vi "SIM Init Special Solver (vector).vi"(4 "Output":dbl[](array[numeric]), 5 "State Index":i32, 6 "State Name":string, 7 "Simulation data":T1={"continuous integrator"=enum."RK 1 (Euler)", "initial time"=0.0, "final time"=0.0, "step size"=0.0, "proposed step size"=0.0, "max step size"=0.0, "min step size"=0.0, "discrete time step"=0.0, "max step ratio"=0.0, "Diag Eval Stage"=enum."Init", "Substep Index"=0, "Timestep Index"=0.0, "simulation time"=0.0, "current timestep base"=0.0, "proposed step time"=0.0, "absolute tolerance"=0.0, "relative tolerance"=0.0, "step accepted?"=FALSE, "step complete?"=FALSE, "Halt?"=FALSE, "reset integrator?"=FALSE, "machine epsilon"=0.0, "min float"=0.0, "error"={"status"=FALSE, "code"=0, "source"=""}, "Method Order"=0, "Finished Late [i-1]"=FALSE, "Discrete step?"=FALSE, "NaN and Inf check?"=FALSE, "Final Timestep Index"=0.0, "(maj+disc)or(init)?"=FALSE, "Full Solver Reset"=TRUE, "Execution Mode"=enum."Simulate to Completion", "check vector sizes?"=FALSE, "solver handles zc?"=FALSE, "Simulation Registry"={"Current Idx"=0, "Node Tags"=[], "Node Headers"=[], "Node Data"=[], "Cont State data"={"inputs"=[], "outputs"=[], "reset"=[], "lower limits"=[], "upper limits"=[], "limit types"=[], "reset types"=[], "initial conditions"=[], "reset I.C."=[], "limited?"=[], "State Names"=[]}, "DiscreteInfo"={"tick period (sec)"=0.0, "time (ticks)"=0, "fire?"=[], "registry"={"period (sec)"=[], "skew (sec)"=[], "period (tick)"=[], "skew (tick)"=[]}, "discrete \nblocks?"=FALSE, "steps per tick"=0.0, "steps to tick"=0.0, "discrete \ntick?"=FALSE}, "Disc State data"={"Disc States"=[], "State Names"=[]}, "Registry Error"={"Error Block ID"=0, "code"=0}, "ZC Indices"=[]}, "variable step solver?"=FALSE, "First Substep?"=FALSE, "Continuous States?"=FALSE} {"min float" format="%.1e"; "proposed step size" format="%.1e"; "proposed step time" format="%.1e"; "max step ratio" format="%.1e"; "min step size" format="%.1e"; "machine epsilon" format="%.1e"; "discrete time step" format="%.1e"; "max step size" format="%.1e"; "current timestep base" format="%.1e"; "final time" format="%.1e"; "simulation time" format="%.1e"; "relative tolerance" format="%.1e"; "absolute tolerance" format="%.1e"; "Substep Index" format="%.1e"; "step size" format="%.1e"; "initial time" format="%.1e"}) -> (0 "Modified Output":dbl[](array[numeric]), 3 "Simulation data out":T1={"continuous integrator"=enum."RK 1 (Euler)", "initial time"=0.0, "final time"=0.0, "step size"=0.0, "proposed step size"=0.0, "max step size"=0.0, "min step size"=0.0, "discrete time step"=0.0, "max step ratio"=0.0, "Diag Eval Stage"=enum."Init", "Substep Index"=0, "Timestep Index"=0.0, "simulation time"=0.0, "current timestep base"=0.0, "proposed step time"=0.0, "absolute tolerance"=0.0, "relative tolerance"=0.0, "step accepted?"=FALSE, "step complete?"=FALSE, "Halt?"=FALSE, "reset integrator?"=FALSE, "machine epsilon"=0.0, "min float"=0.0, "error"={"status"=FALSE, "code"=0, "source"=""}, "Method Order"=0, "Finished Late [i-1]"=FALSE, "Discrete step?"=FALSE, "NaN and Inf check?"=FALSE, "Final Timestep Index"=0.0, "(maj+disc)or(init)?"=FALSE, "Full Solver Reset"=TRUE, "Execution Mode"=enum."Simulate to Completion", "check vector sizes?"=FALSE, "solver handles zc?"=FALSE, "Simulation Registry"={"Current Idx"=0, "Node Tags"=[], "Node Headers"=[], "Node Data"=[], "Cont State data"={"inputs"=[], "outputs"=[], "reset"=[], "lower limits"=[], "upper limits"=[], "limit types"=[], "reset types"=[], "initial conditions"=[], "reset I.C."=[], "limited?"=[], "State Names"=[]}, "DiscreteInfo"={"tick period (sec)"=0.0, "time (ticks)"=0, "fire?"=[], "registry"={"period (sec)"=[], "skew (sec)"=[], "period (tick)"=[], "skew (tick)"=[]}, "discrete \nblocks?"=FALSE, "steps per tick"=0.0, "steps to tick"=0.0, "discrete \ntick?"=FALSE}, "Disc State data"={"Disc States"=[], "State Names"=[]}, "Registry Error"={"Error Block ID"=0, "code"=0}, "ZC Indices"=[]}, "variable step solver?"=FALSE, "First Substep?"=FALSE, "Continuous States?"=FALSE} {"min float" format="%.1e"; "proposed step size" format="%.1e"; "proposed step time" format="%.1e"; "max step ratio" format="%.1e"; "min step size" format="%.1e"; "machine epsilon" format="%.1e"; "discrete time step" format="%.1e"; "max step size" format="%.1e"; "current timestep base" format="%.1e"; "final time" format="%.1e"; "simulation time" format="%.1e"; "relative tolerance" format="%.1e"; "absolute tolerance" format="%.1e"; "Substep Index" format="%.1e"; "step size" format="%.1e"; "initial time" format="%.1e"})   [LabVIEW 2017]
uses:
  <vilib>/Simulation/Implementation/Shared/SIM simulation data.ctl
  <vilib>/Simulation/Implementation/Shared/SIM integration method.ctl
  <vilib>/Simulation/Implementation/Shared/SIM diagram eval stage.ctl
  <vilib>/Simulation/Implementation/Shared/SIMSCR Execution Mode.ctl
  <vilib>/Simulation/Implementation/Shared/SIM Registry.llb/SIM Simulation Registry.ctl
  <vilib>/Simulation/Implementation/Shared/SIM Registry.llb/SIM Registry Node Header.ctl
  <vilib>/Simulation/Implementation/Shared/SIM Registry.llb/SIM Registry Node Record.ctl
  <vilib>/Simulation/Implementation/Shared/SIM trigger type.ctl
  <vilib>/Simulation/Implementation/Shared/SIM solver state data.ctl
  <vilib>/Simulation/Implementation/Shared/SIM limit type.ctl
  <vilib>/Simulation/Implementation/Shared/SIM discrete data.ctl
  <vilib>/Simulation/Implementation/Shared/SIM Discrete state data.ctl
  <vilib>/Simulation/Implementation/Shared/SIM Registry.llb/SIM Simulation Registry Error.ctl
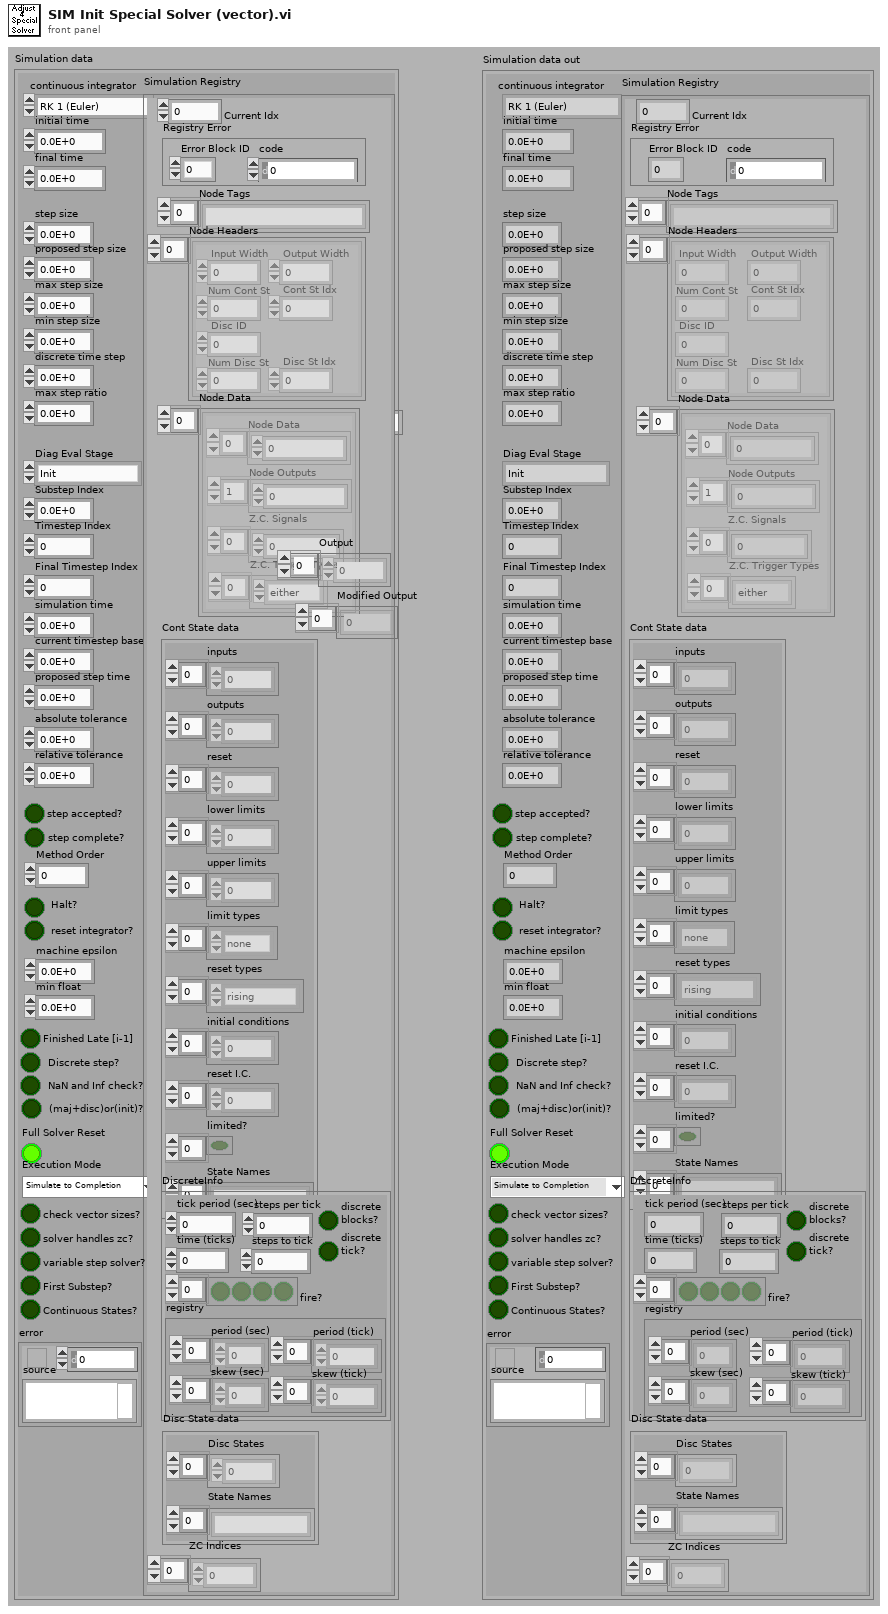
[diagram p1: front panel]
types:
  T1 = typedef "SIM simulation data.ctl" = cluster{"continuous integrator":T2, "initial time":dbl, "final time":dbl, "step size":dbl, "proposed step size":dbl, "max step size":dbl, "min step size":dbl, "discrete time step":dbl, "max step ratio":dbl, "Diag Eval Stage":T3, "Substep Index":i32, "Timestep Index":dbl, "simulation time":dbl, "current timestep base":dbl, "proposed step time":dbl, "absolute tolerance":dbl, "relative tolerance":dbl, "step accepted?":bool, "step complete?":bool, "Halt?":bool, "reset integrator?":bool, "machine epsilon":dbl, "min float":dbl, "error":errorcluster, "Method Order":u32, "Finished Late [i-1]":bool, "Discrete step?":bool, "NaN and Inf check?":bool, "Final Timestep Index":dbl, "(maj+disc)or(init)?":bool, "Full Solver Reset":bool, "Execution Mode":T4, "check vector sizes?":bool, "solver handles zc?":bool, "Simulation Registry":T5, "variable step solver?":bool, "First Substep?":bool, "Continuous States?":bool}
  T2 = typedef "SIM integration method.ctl" = enum16{"RK 1 (Euler)", "Linearizer", "State Query", "Trim Eval", "Adams", "RK 3", "RK 4", "RK 45", "BDF", "RK 2", "RK 23", "Rosenbrock", "Discrete States Only"}
  T3 = typedef "SIM diagram eval stage.ctl" = enum16{"Init", "Minor Substep", "Major Substep", "Final"}
  T4 = typedef "SIMSCR Execution Mode.ctl" = enum16{"Simulate to Completion", "Single Time-Step Simulation (Fixed Step Only)"}
  T5 = typedef "SIM Simulation Registry.ctl" = cluster{"Current Idx":i32, "Node Tags":string[], "Node Headers":T6[], "Node Data":T7[], "Cont State data":T9, "DiscreteInfo":T11, "Disc State data":T12, "Registry Error":T13, "ZC Indices":i32[]}
  T6 = typedef "SIM Registry Node Header.ctl" = cluster{"Input Width":i32, "Disc ID":i32, "Num Cont St":i32, "Cont St Idx":i32, "Num Disc St":i32, "Disc St Idx":i32, "Output Width":i32}
  T7 = typedef "SIM Registry Node Record.ctl" = cluster{"Node Data":dbl[], "Node Outputs":dbl[], "Z.C. Signals":dbl[], "Z.C. Trigger Types":T8[]}
  T8 = typedef "SIM trigger type.ctl" = enum16{"rising", "falling", "either", "none"}
  T9 = typedef "SIM solver state data.ctl" = cluster{"inputs":dbl[], "outputs":dbl[], "reset":dbl[], "lower limits":dbl[], "upper limits":dbl[], "limit types":T10[], "reset types":T8[], "initial conditions":dbl[], "reset I.C.":dbl[], "limited?":bool[], "State Names":string[]}
  T10 = typedef "SIM limit type.ctl" = enum16{"upper", "lower", "both", "none"}
  T11 = typedef "SIM discrete data.ctl" = cluster{"tick period (sec)":dbl, "time (ticks)":i32, "fire?":bool[], "registry":cluster{"period (sec)":dbl[], "skew (sec)":dbl[], "period (tick)":i32[], "skew (tick)":i32[]}, "discrete \nblocks?":bool, "steps per tick":dbl, "steps to tick":dbl, "discrete \ntick?":bool}
  T12 = typedef "SIM Discrete state data.ctl" = cluster{"Disc States":dbl[], "State Names":string[]}
  T13 = typedef "SIM Simulation Registry Error.ctl" = cluster{"Error Block ID":i32, "code":i32}
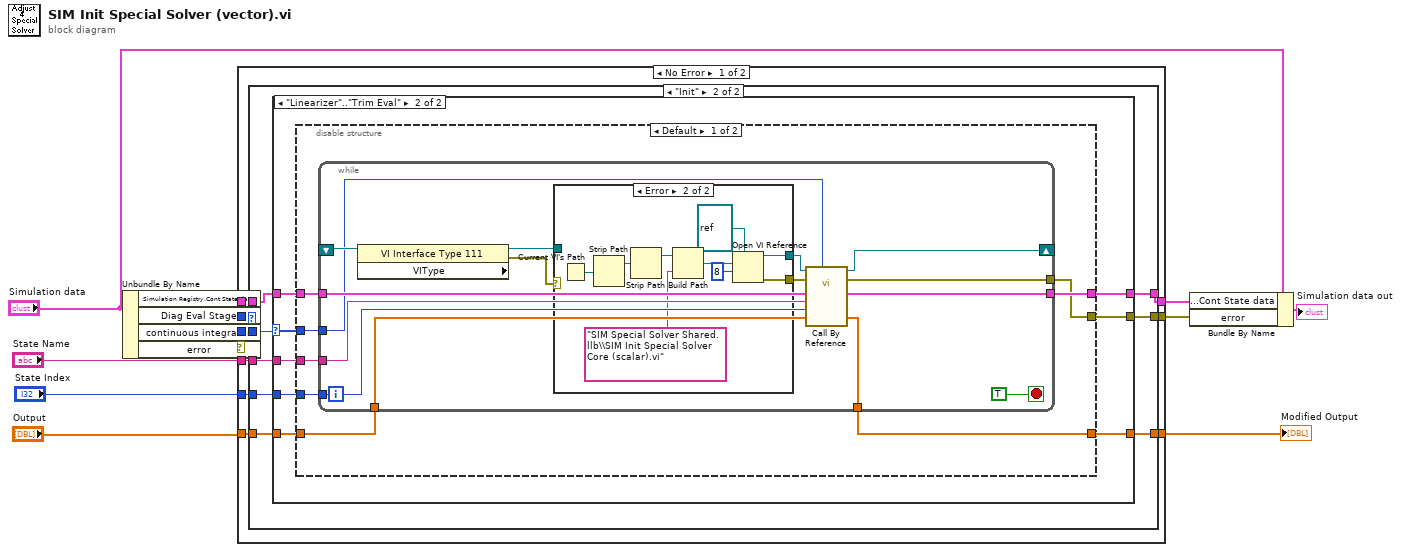
[diagram p0: block diagram]
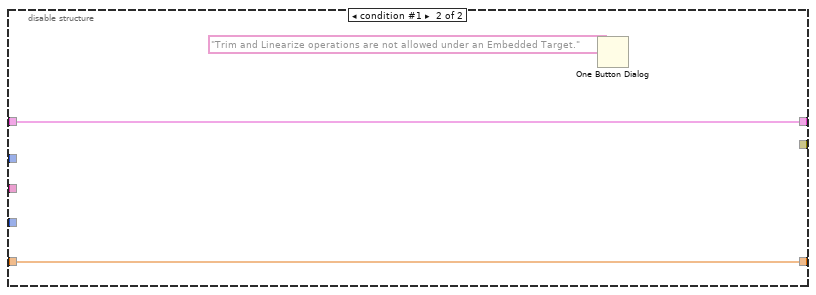
[diagram p5: hidden frame]
diagram:
  n1 = Unbundle By Name("Simulation data") -> ("Simulation Registry.Cont State data"=w10:T9, "Diag Eval Stage"=w12:T3, "continuous integrator"=w11:T2, "error"=w8:errorcluster)
  n2 = case shown="No Error" w8 {
    selector: w8 -> [_ w79]
    tunnel: "State Name" -> [w21 _]
    tunnel: "State Index" -> [w20 _]
    tunnel: w12 -> [w19 _]
    tunnel: "Output" -> [w18 _]
    tunnel: [w17 _] -> w1
    tunnel: w11 -> [w16 _]
    tunnel: w10 -> [w15 w80]
    tunnel: [w14 w80] -> w9
    tunnel: [w13 w79] -> w7
    frame No Error {
      n3 = case shown="\"Init\"" w19 {
        tunnel: w21 -> [_ w28]
        tunnel: w20 -> [_ w29]
        tunnel: w15 -> [w23 w31]
        tunnel: [w23 w27] -> w14
        tunnel: w18 -> [w22 w30]
        tunnel: [w22 w26] -> w17
        tunnel: w16 -> [_ w25]
        tunnel: [_ w24] -> w13
        frame Default {
        }
        frame "Init" {
          n4 = case shown="\"Linearizer\"..\"Trim Eval\"" w25 {
            selector: w25 -> [_ w35]
            tunnel: w31 -> [w32 w41]
            tunnel: w30 -> [w33 w40]
            tunnel: w29 -> [_ w36]
            tunnel: w28 -> [_ w39]
            tunnel: [w32 w37] -> w27
            tunnel: [w33 w38] -> w26
            tunnel: [_ w34] -> w24
            frame Default {
            }
            frame "Linearizer".."Trim Eval" {
              n5 = disable-structure shown="Default" {
                disable-tunnel: w41 -> [w49 w78]
                disable-tunnel: w40 -> [w48 w77]
                disable-tunnel: w39 -> [w47 _]
                disable-tunnel: [w46 w77] -> w38
                disable-tunnel: [w45 w78] -> w37
                disable-tunnel: w36 -> [w44 _]
                disable-tunnel: w35 -> [w43 _]
                disable-tunnel: [w42 _] -> w34
                frame condition #0 (active) {
                  n6 = while {
                    tunnel: w49 -> [w60]
                    tunnel: w48 -> [w57]
                    tunnel: w47 -> [w59]
                    tunnel: [w56] -> w46
                    tunnel: [w52] -> w45
                    tunnel: w44 -> [w58]
                    shift-right: [w55] -> _
                    shift-left: _ -> [w63]
                    tunnel: w43 -> [w51]
                    tunnel: [w50] -> w42
                    stop <- TRUE stop-if-true
                    n7 = property class="VI Interface Type 111" props=["VIType"](reference=w63) -> (reference out=w54:refnum<vi>, error out=w61:errorcluster)  [unwired: 1 in, 1 out]
                    n8 = case shown="Error" w61 {
                      selector: w61 -> [w66 _]
                      tunnel: [w66 w75] -> w64
                      tunnel: [w65 w69] -> w53
                      tunnel: w54 -> [w65 _]
                      frame No Error {
                      }
                      frame Error {
                        n9 = Current VI's Path() -> (path=w74:path)
                        n10 = Strip Path(path=w74) -> (stripped path=w68:path)  [unwired: 1 out]
                        n11 = Strip Path(path=w68) -> (stripped path=w67:path)  [unwired: 1 out]
                        n12 = Build Path(base path=w67, name or relative path="SIM Special Solver Shared.llb\\SIM Init Special Solver Core (scalar).vi") -> (appended path=w72:path)
                        n13 = Open VI Reference(type specifier VI Refnum (for type only)=refnum<vi> refnum, vi path=w72, options=8) -> (vi reference=w69:refnum<vi>, error out=w75:errorcluster)  [unwired: 1 in, 2 out]
                      }
                    }
                    n14 = call-by-ref "?"(reference=w53, error in=w64, "continuous integrator"=w51, "Output"=w57, "State Index"=w58, "State Name"=w59, "State data in"=w60) -> (reference out=w55:refnum<vi>, error out=w50:errorcluster, "Modified Output"=w56:dbl[], "State data"=w52:T9)  [unwired: 5 in]
                  }
                }
                frame condition #1 {
                  n15 = One Button Dialog(message="Trim and Linearize operations are not allowed under an Embedded Target.") -> ()  [unwired: 1 in, 1 out]
                }
              }
            }
          }
        }
      }
    }
    frame Error {
    }
  }
  "Modified Output" <- w1
  n16 = Bundle By Name(cluster="Simulation data", "Simulation Registry.Cont State data"=w9, "error"=w7) -> (→"Simulation data out":T1)
